vi "Berechnung_U_Mess.vi"(7 "Oszi-Channel (1)":T1=1.0 min=1.0 max=4.0 step=1.0 format="%#_1g", 8 "Error In (No Error)":errorcluster, 9 "Faktor (1)":dbl=1.0, 10 "Messdaten_Array_1D":dbl[](array[numeric]), 11 "VISA Name OZ In (OZ)":refnum<visa-resource-name>="USB0::0x0957::0x179B::MY54313507::INSTR") -> (0 "Error Out":errorcluster, 1 "Output Array":dbl[](array[numeric]), 3 "VISA Name OZ Out":refnum<visa-resource-name>="USB0::0x0957::0x179B::MY54313507::INSTR")   [LabVIEW 2016]
doc: "Berechnet die wahren Spannungswerte welche vom Oszi gemessen wurden.\nDer Faktor wird optional am Ende des Berechnungsalgorithmus auf das Ergebnis multipliziert."
uses:
  controls/Oszi_KanalInfo.ctl
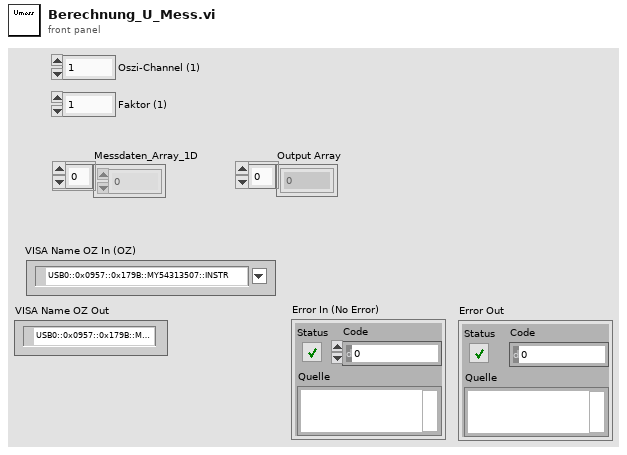
[diagram p1: front panel]
types:
  T1 = typedef "Oszi_KanalInfo.ctl" = dbl
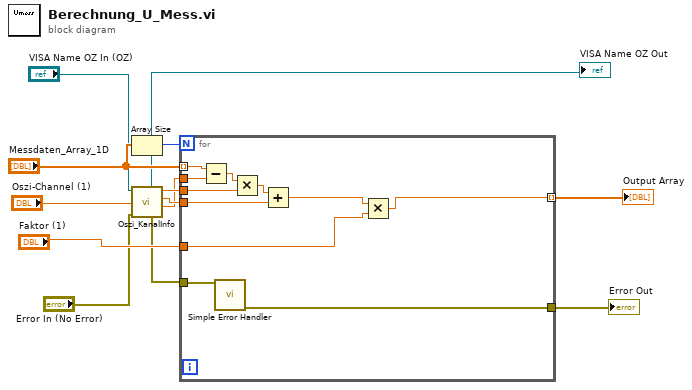
[diagram p0: block diagram]
diagram:
  n1 = Array Size(array="Messdaten_Array_1D") -> (size(s)=w11:i32)
  n2 = call "Oszi_KanalInfo.vi"("Error In (No Error)"="Error In (No Error)", "Oszi-Channel (1)"="Oszi-Channel (1)", "VISA Name OZ In (OZ)"="VISA Name OZ In (OZ)") -> ("YREFerence"=w8:dbl, "YORigin"=w9:dbl, "YINcrement"=w10:dbl, "Error Out"=w3:errorcluster, "VISA Name OZ Out"=→"VISA Name OZ Out":refnum<visa-resource-name>)  [unwired: 3 in, 1 out]
  n3 = for {
    N: w11 -> [_]
    tunnel: "Messdaten_Array_1D" -> [w22] mode=indexing
    tunnel: [w15] -> w13 mode=indexing
    tunnel: w10 -> [w21]
    tunnel: w9 -> [w20]
    tunnel: w8 -> [w19]
    tunnel: w3 -> [w18]
    tunnel: [w17] -> w7
    tunnel: "Faktor (1)" -> [w14]
    n4 = Subtract(x=w22, y=w19) -> (x-y=w24:dbl)
    n5 = call <vilib>:"Simple Error Handler.vi"("error in (no error)"=w18) -> ("error out"=w17:errorcluster)  [unwired: 4 in, 4 out]
    n6 = Multiply(x=w24, y=w21) -> (x*y=w23:dbl)
    n7 = Add(x=w23, y=w20) -> (x+y=w16:dbl)
    n8 = Multiply(x=w16, y=w14) -> (x*y=w15:dbl)
  }
  "Output Array" <- w13
  "Error Out" <- w7
